vi "New Child.vi"(7 "Value Type (Object)":T1=enum."Object", 8 "error in (no error)":errorcluster, 9 "Child Name":string, 10 "Parent":refnum<class "Config Element.lvclass">, 11 "Config Manager in":refnum<class "Config Manager.lvclass">) -> (0 "error out":errorcluster, 1 "New Child":refnum<class "Config Element.lvclass">, 3 "Config Manager out":refnum<class "Config Manager.lvclass">)   [LabVIEW 2023, in "CDM-Config.lvlib" / "Config Manager.lvclass"]
doc: "Creates a new element directly under the specified parent element with the specified name. All direct children of an element must have unique names. Additionally, children cannot be named \"Meta\" as that is reserved for persisting and loading configs."
uses:
  Config Manager.lvclass
  Config Element/Config Element.lvclass
  Value Type.ctl
  Config Manager.lvclass/Config Manager.ctl
  CDM-Config.lvlib
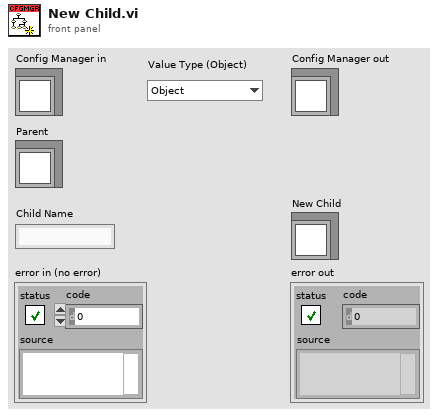
[diagram p1: front panel]
types:
  T1 = typedef "CDM-Config.lvlib/Value Type.ctl" = enum16{"String", "Number", "Bool", "Object", "Array"}
  T2 = typedef "CDM-Config.lvlib/Config Manager.lvclass/Ref Data.ctl" = cluster{"Elements":refnum<class "Config Element.lvclass">[], "Hierarchy Map":map{string[], i32}, "Element Map":map{refnum<class "Config Element.lvclass">, i32}}
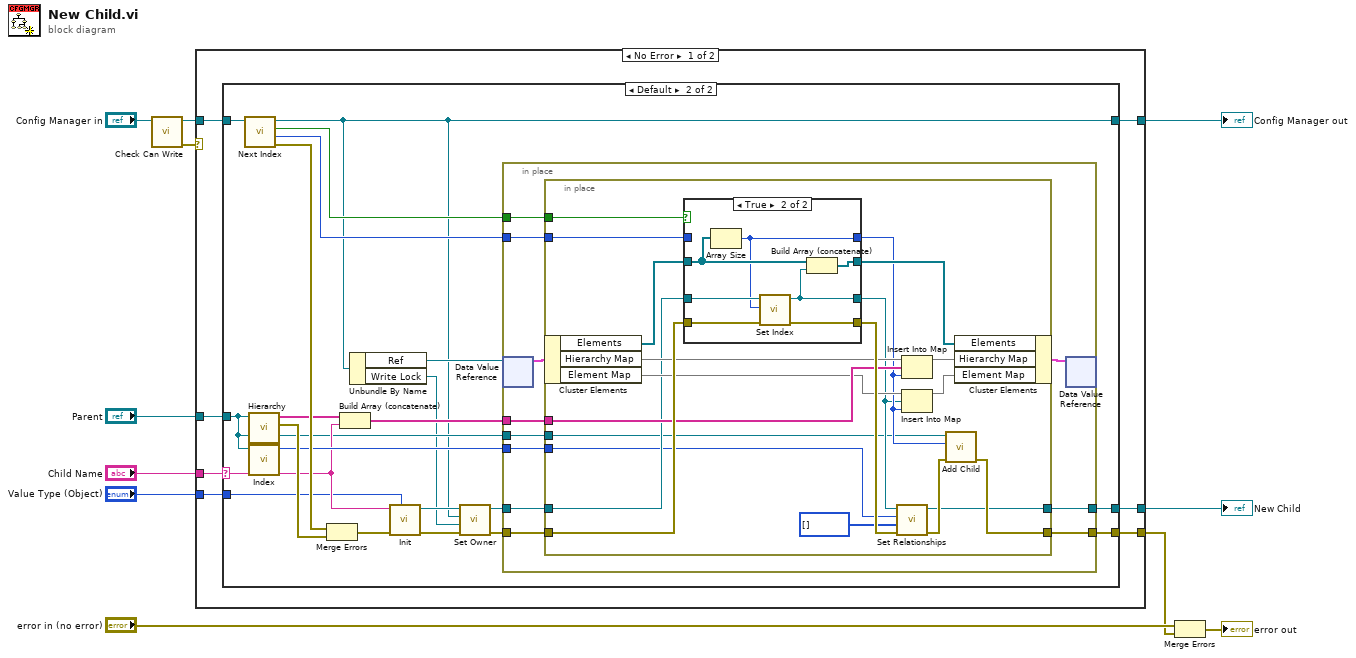
[diagram p0: block diagram]
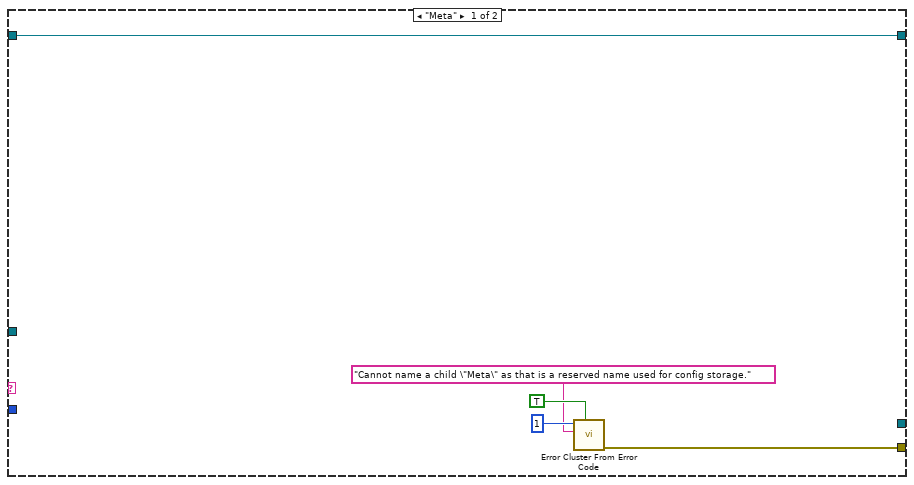
[diagram p2: hidden frame]
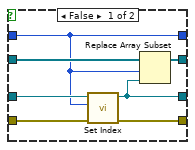
[diagram p3: hidden frame]
diagram:
  n1 = call "Check Can Write.vi"("Config Manager in"="Config Manager in") -> ("error out"=w1:errorcluster, "Config Manager out"=w2:refnum<class "Config Manager.lvclass">)  [unwired: 9 in]
  n2 = case shown="No Error" w1 {
    selector: w1 -> [_ w90]
    tunnel: "Parent" -> [w18 _]
    tunnel: "Child Name" -> [w17 _]
    tunnel: w2 -> [w16 w91]
    tunnel: [w15 _] -> w7
    tunnel: [w14 w91] -> w6
    tunnel: [w13 w90] -> w4
    tunnel: "Value Type (Object)" -> [w12 _]
    frame No Error {
      n3 = case shown="Default" w17 {
        selector: w17 -> [_ w32]
        tunnel: w18 -> [_ w30]
        tunnel: w16 -> [w23 w40]
        tunnel: [_ w35] -> w15
        tunnel: [w23 w28] -> w14
        tunnel: [w19 w33] -> w13
        tunnel: w12 -> [_ w31]
        frame "Meta" {
          n4 = call <vilib>:"Error Cluster From Error Code.vi"("show call chain? (False)"=TRUE, "error message (\"\")"="Cannot name a child \"Meta\" as that is a reserved name used for config storage.", "error code (0)"=1) -> ("error out"=w19:errorcluster)  [unwired: 6 in]
        }
        frame Default {
          n5 = call "Next Index.vi"("Config Manager in"=w40) -> ("error out"=w44:errorcluster, "Index"=w37:i32, "Add to End"=w36:bool, "Config Manager out"=w28:refnum<class "Config Manager.lvclass">)  [unwired: 7 in]
          n6 = call "Hierarchy.vi"("Config Element in"=w30) -> ("error out"=w43:errorcluster, "Hierarchy"=w42:string[])  [unwired: 9 in]
          n7 = call "Index.vi"("Config Element in"=w30) -> ("Index"=w38:i32)  [unwired: 9 in, 1 out]
          n8 = Merge Errors(w44, w43) -> (w34:errorcluster)
          n9 = Build Array (concatenate)(w42, w32) -> (w39:string[])
          n10 = Unbundle By Name(w28) -> ("Ref"=w41:refnum<data-value>, "Write Lock"=w27:refnum<notifier>)
          n11 = call "Init.vi"("Value Type"=w31, "error in (no error)"=w34, "Name"=w32) -> ("error out"=w26:errorcluster, "Config Element out"=w29:refnum<class "Config Element.lvclass">)  [unwired: 7 in]
          n12 = call "Set Owner.vi"("error in (no error)"=w26, "Write Lock"=w27, "Owner"=w28, "Config Element in"=w29) -> ("error out"=w25:errorcluster, "Config Element out"=w24:refnum<class "Config Element.lvclass">)  [unwired: 6 in]
          n13 = in-place {
            in-place-border: w24 -> [w53]
            in-place-border: w39 -> [w52]
            in-place-border: [w51] -> w35
            in-place-border: w38 -> [w50]
            in-place-border: w37 -> [w49]
            in-place-border: w36 -> [w48]
            in-place-border: w25 -> [w47]
            in-place-border: [w46] -> w33
            in-place-border: w30 -> [w45]
            n14 = in-place-dvr #1(w41) -> (w55:T2)  [unwired: 1 out]
            n15 = in-place {
              in-place-border: w53 -> [w65]
              in-place-border: w52 -> [w69]
              in-place-border: [w61] -> w51
              in-place-border: w50 -> [w60]
              in-place-border: w49 -> [w63]
              in-place-border: w48 -> [w62]
              in-place-border: w47 -> [w75]
              in-place-border: [w72] -> w46
              in-place-border: w45 -> [w56]
              n16 = in-place-cluster #2(w55) -> ("Elements"=w71:refnum<class "Config Element.lvclass">[], "Hierarchy Map"=w70:map{string[], i32}, "Element Map"=w68:map{refnum<class "Config Element.lvclass">, i32})
              n17 = case shown="True" w62 {
                tunnel: w71 -> [w82 w88]
                tunnel: w65 -> [w80 w87]
                tunnel: [w81 w89] -> w64
                tunnel: [w79 w85] -> w58
                tunnel: w63 -> [w79 _]
                tunnel: [w78 w86] -> w57
                tunnel: w75 -> [w77 w84]
                tunnel: [w76 w83] -> w74
                frame False {
                  n18 = call "Set Index.vi"("error in (no error)"=w77, "Index"=w79, "Config Element in"=w80) -> ("error out"=w76:errorcluster, "Config Element out"=w78:refnum<class "Config Element.lvclass">)  [unwired: 7 in]
                  n19 = Replace Array Subset(array=w82, new element=w78, index=w79) -> (w81:refnum<class "Config Element.lvclass">[])
                }
                frame True {
                  n20 = Array Size(array=w88) -> (size(s)=w85:i32)
                  n21 = call "Set Index.vi"("error in (no error)"=w84, "Index"=w85, "Config Element in"=w87) -> ("error out"=w83:errorcluster, "Config Element out"=w86:refnum<class "Config Element.lvclass">)  [unwired: 7 in]
                  n22 = Build Array (concatenate)(w88, w86) -> (w89:refnum<class "Config Element.lvclass">[])
                }
              }
              n23 = call "Set Relationships.vi"("error in (no error)"=w74, "Children"=i32[] [], "Parent"=w60, "Config Element in"=w57) -> ("error out"=w73:errorcluster, "Config Element out"=w61:refnum<class "Config Element.lvclass">)  [unwired: 6 in]
              n24 = Insert Into Map(map in=w70, key=w69, value=w58) -> (map out=w67:map{string[], i32})  [unwired: 2 out]
              n25 = Insert Into Map(map in=w68, key=w57, value=w58) -> (map out=w66:map{refnum<class "Config Element.lvclass">, i32})  [unwired: 2 out]
              n26 = call "Add Child.vi"("error in (no error)"=w73, "Child"=w58, "Config Element in"=w56) -> ("error out"=w72:errorcluster)  [unwired: 7 in, 1 out]
              n27 = in-place-cluster #2("Elements"=w64, "Hierarchy Map"=w67, "Element Map"=w66) -> (w54:T2)
            }
            n28 = in-place-dvr #1(w54) -> ()  [unwired: 2 out]
          }
        }
      }
    }
    frame Error {
    }
  }
  "Config Manager out" <- w6
  "New Child" <- w7
  n29 = Merge Errors("error in (no error)", w4) -> (→"error out":errorcluster)
